vi "Create.vi"() -> (8 "SAM":refnum<class "SAM.lvclass">)   [LabVIEW 2020, in "SAM.lvclass"]
uses:
  SAM.lvclass
  D:/Development/epl-vi-lib/Signal Synthesis VIs/4th Generation/Classes/Modulations/AM/AM.lvclass
  SAM.lvclass/SAM.ctl
  AM/AM.lvclass/AM.ctl
  Write Frequency (Hz).vi
  AM/Write Depth (0-1).vi
  AM/Write Correct level .vi
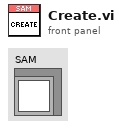
[diagram p1: front panel]
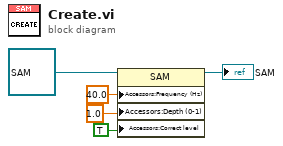
[diagram p0: block diagram]
diagram:
  n1 = property class="SAM"(reference=refnum<class "SAM.lvclass"> refnum ("SAM"), "Accessors:Frequency (Hz)"=40.0 ("Frequency (Hz)"), "Accessors:Depth (0-1)"=1.0 ("Serialized.Depth (0-1)"), "Accessors:Correct level "=TRUE ("Correct level")) -> (reference out=→"SAM":refnum<class "SAM.lvclass">)  [unwired: 1 in, 1 out]
